vi "To 2D String Tree Data.vi"(10 "2D String":string[][](array[string])) -> (3 "2D String Tree Data":refnum<class "2D String.lvclass">)   [LabVIEW 2020, in "NI_VIAnCFGDataStructure.lvlib" / "2D String.lvclass"]
doc: "Convert a 2D String value to Tree Data type."
uses:
  <vilib>/addons/analyzer/VIAnCFGDataStructure/Data Types/2D String/2D String.lvclass
  <vilib>/addons/analyzer/VIAnCFGDataStructure/Data Types/2D String/2D String.lvclass/2D String.ctl
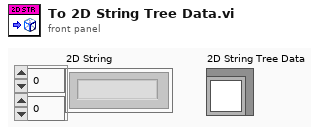
[diagram p1: front panel]
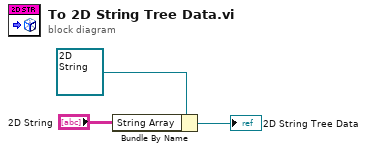
[diagram p0: block diagram]
diagram:
  n1 = Bundle By Name(cluster=refnum<class "2D String.lvclass"> refnum ("Tree API.lvlib:2D String.lvclass"), "String Array"="2D String") -> (→"2D String Tree Data":refnum<class "2D String.lvclass">)
